vi "CSTK_Icon_Creator_Dialog.vi"() -> ()   [LabVIEW 2015, in "CSTK_Icon Creator.lvlib"]
uses:
  CSTK_Icon Creator.lvlib
  <vilib>/Utility/miscctls.llb/LVBoundsTypeDef.ctl
  <vilib>/picture/picture.llb/imagedata.ctl
  CSTK_Icon_Creator_Template.ctl
  user32.dll
panel:
  in  "Shutdown":bool
  in  "Minimize":bool
  in  "字体":enum16{"Small Fonts", "6px2bus"}(ring)
  in  "偏移":i8(slide) caption="0" scale=-16.0..16.0
  in  "LOGO":u16(ring)
  in  "保存图标按钮":bool
  in  "生成图标按钮":bool
  in  "主体背景色":u32(colorbox)=16777215
  in  "标题背景色":u32(colorbox)=16777215
  in  "字体颜色":u32(colorbox)
  in  "标题字符":string
  out "4#":picture
  out "3#":picture
  out "2#":picture
  out "1#":picture
  # "Icon Creator"
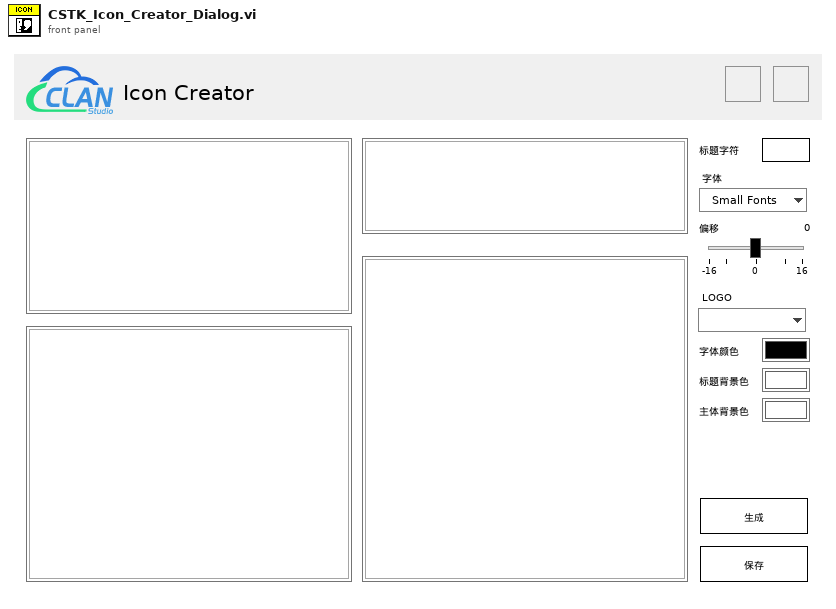
[diagram p1: front panel]
types:
  T1 = enum32{"Invalid", "Standard", "Closed", "Hidden", "Minimized", "Maximized"}
  T2 = typedef "imagedata.ctl" = cluster{"image type":i32, "image depth":i32, "image":u8[], "mask":u8[], "colors":u32[], "Rectangle":cluster{"left":i16, "top":i16, "right":i16, "bottom":i16}}
  T3 = typedef "LVBoundsTypeDef.ctl" = cluster{"Width":u32, "Height":u32}
  T4 = typedef "CSTK_Icon Creator.lvlib/CSTK_Icon_Creator_Template.ctl" = enum16{"1#", "2#", "3#", "4#", "Ctl"}
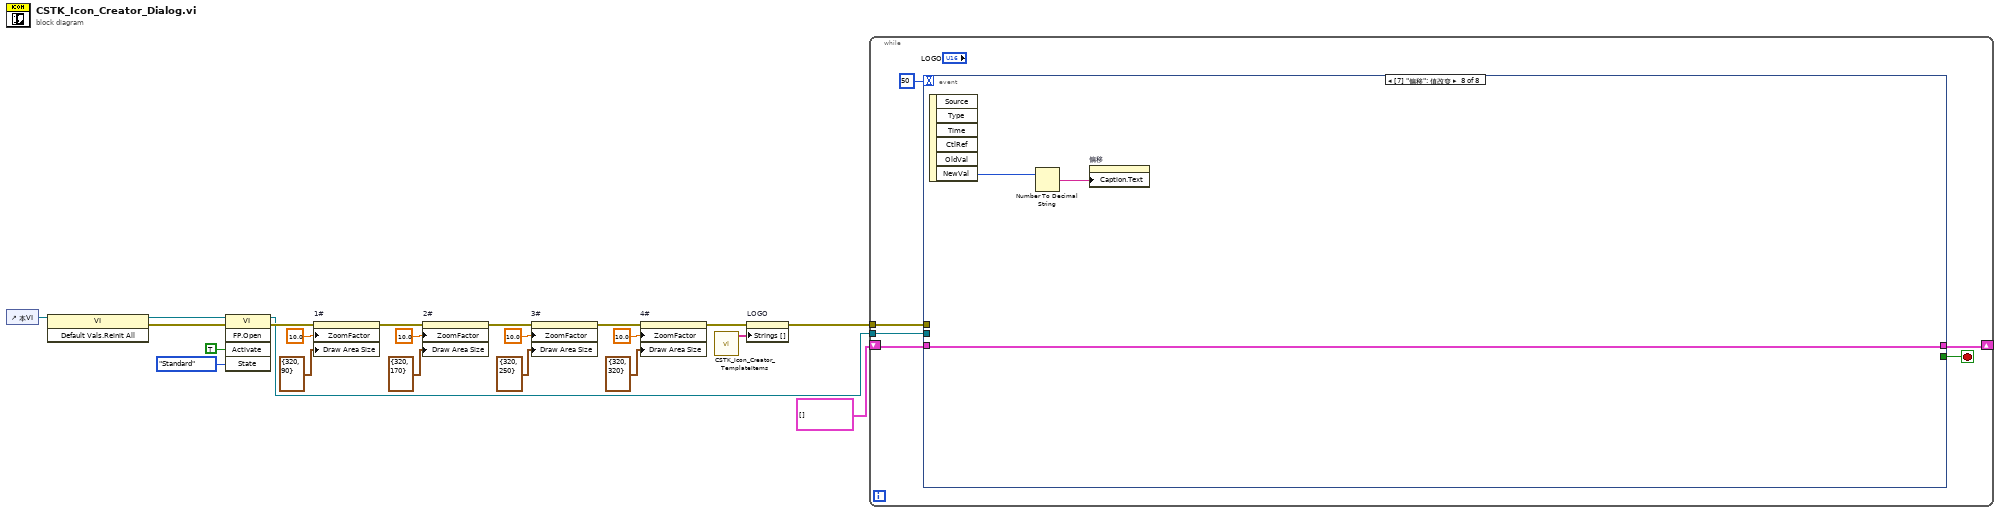
[diagram p0: block diagram]
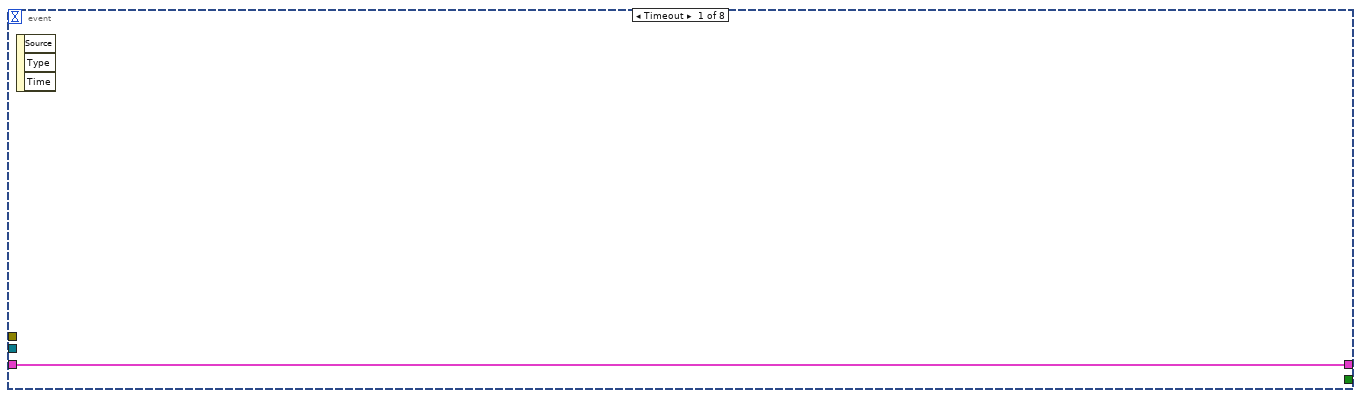
[diagram p2: hidden frame]
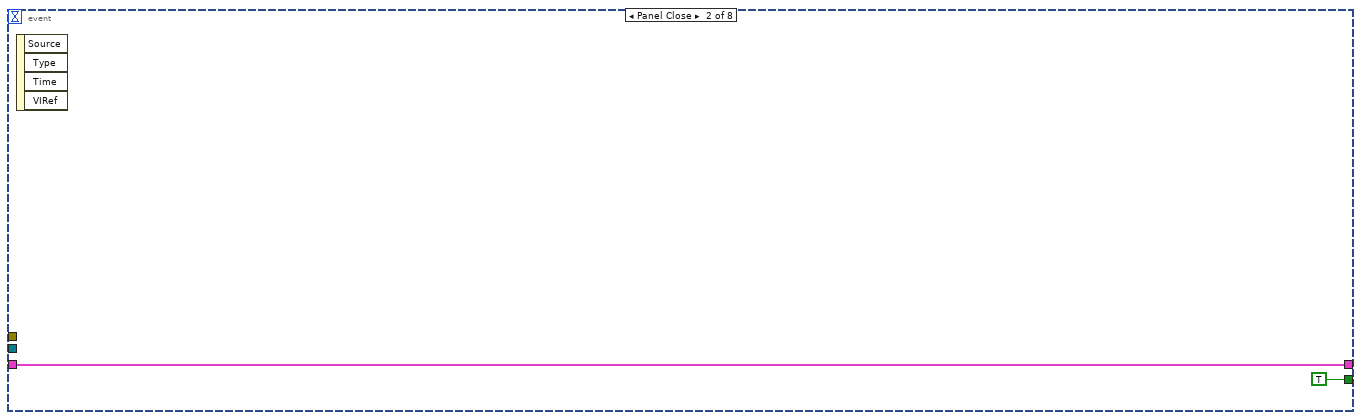
[diagram p3: hidden frame]
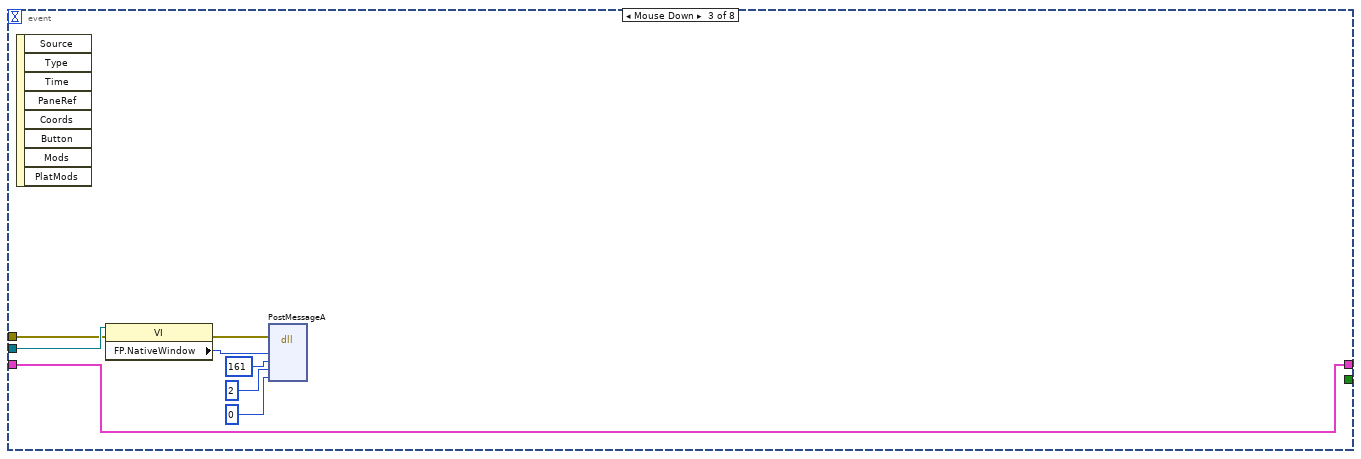
[diagram p4: hidden frame]
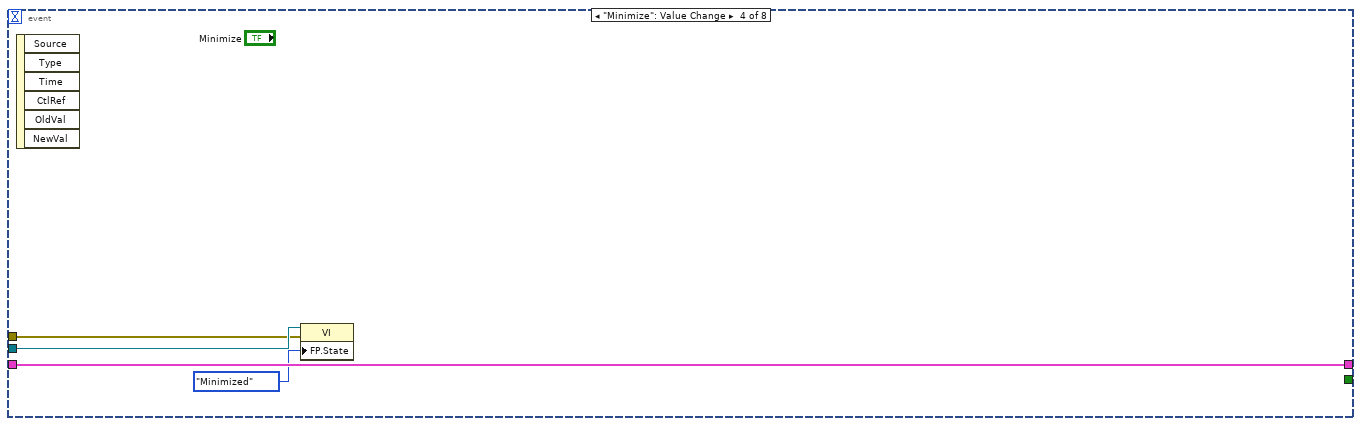
[diagram p5: hidden frame]
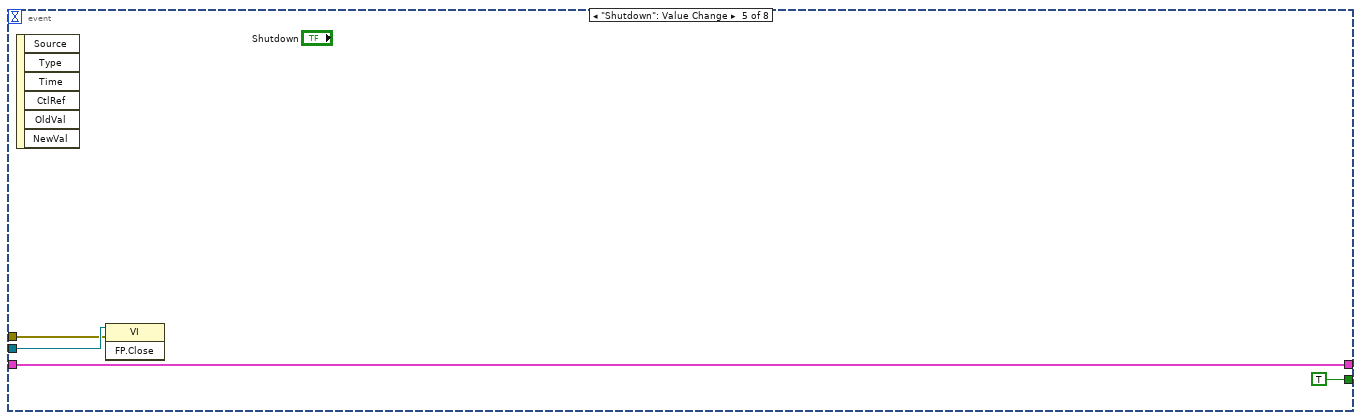
[diagram p6: hidden frame]
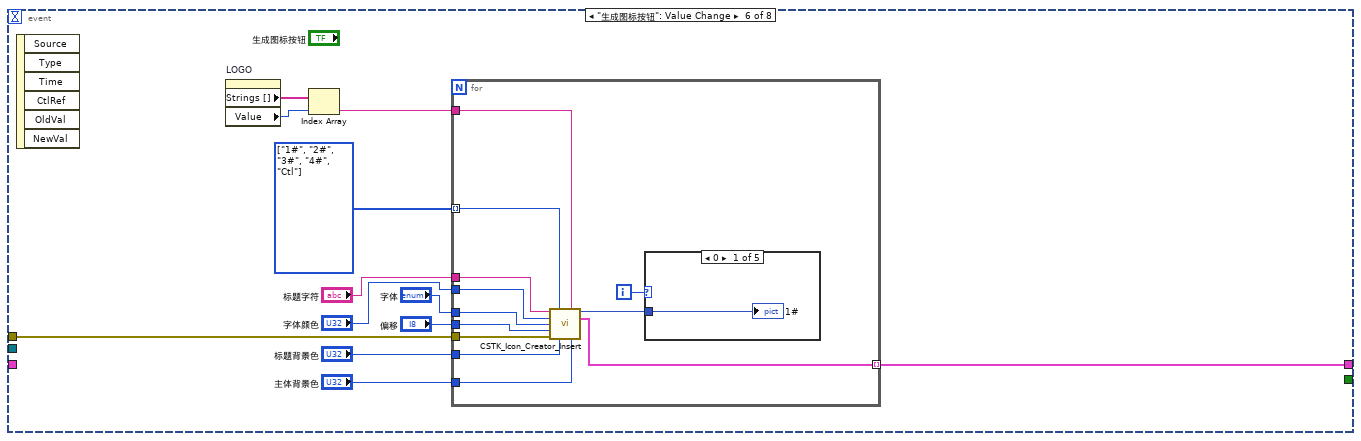
[diagram p7: hidden frame]
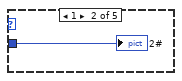
[diagram p8: hidden frame]
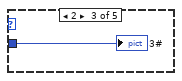
[diagram p9: hidden frame]
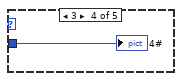
[diagram p10: hidden frame]
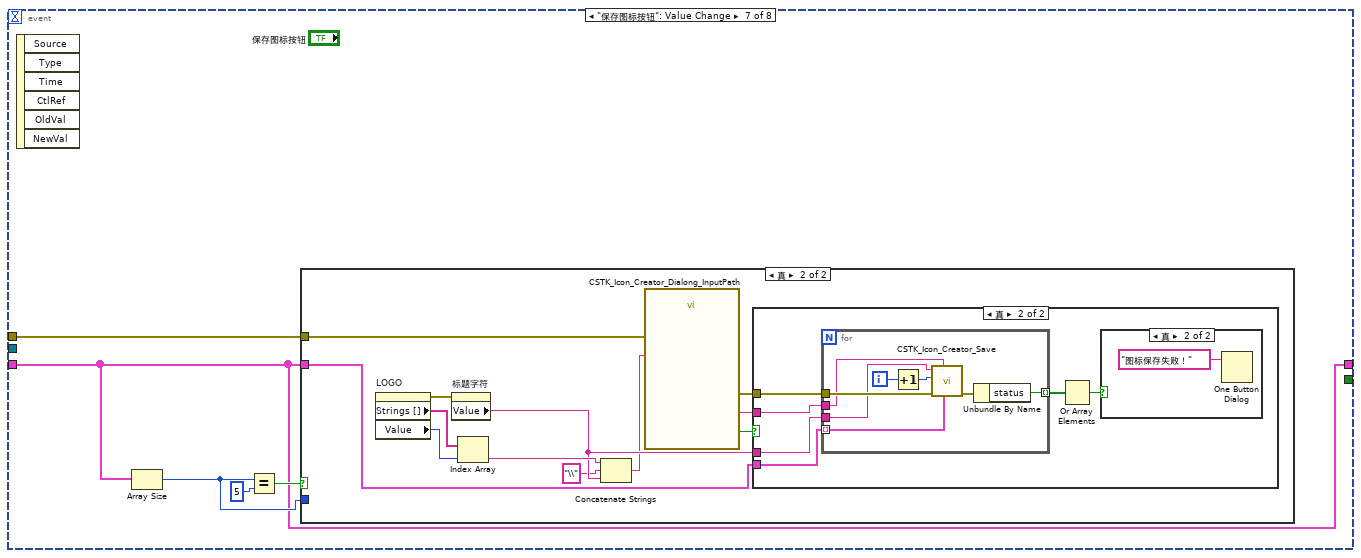
[diagram p12: hidden frame]
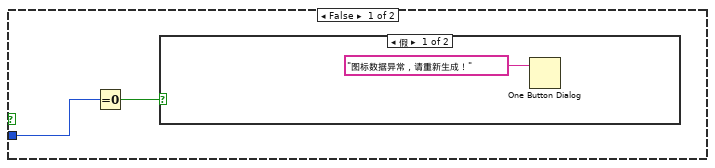
[diagram p13: hidden frame]
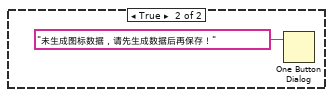
[diagram p14: hidden frame]
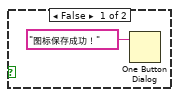
[diagram p16: hidden frame]
diagram:
  n1 = control-ref of="本VI"() -> (w10:refnum<vi>)
  n2 = invoke class="VI" method="Default Vals.Reinit All"(reference=w10) -> (reference out=w8:refnum<vi>, error out=w9:errorcluster)  [unwired: 2 in, 1 out]
  n3 = invoke class="VI" method="FP.Open"(reference=w8, error in=w9, "Activate"=TRUE ("激活？"), "State"=T1."Standard" ("状态")) -> (reference out=w1:refnum<vi>, error out=w7:errorcluster)  [unwired: 1 in, 3 out]
  n4 = property on="1#" class="Pict"(error in=w7, "ZoomFactor"=sgl 10.0 ("缩放因子"), "Draw Area Size"=T3 {"Width"=320, "Height"=90} ("绘图区域大小")) -> (error out=w18:errorcluster)  [unwired: 1 in, 1 out]
  n5 = property on="2#" class="Pict"(error in=w18, "ZoomFactor"=sgl 10.0 ("缩放因子"), "Draw Area Size"=T3 {"Width"=320, "Height"=170} ("绘图区域大小")) -> (error out=w15:errorcluster)  [unwired: 1 in, 1 out]
  n6 = property on="3#" class="Pict"(error in=w15, "ZoomFactor"=sgl 10.0 ("缩放因子"), "Draw Area Size"=T3 {"Width"=320, "Height"=250} ("绘图区域大小")) -> (error out=w12:errorcluster)  [unwired: 1 in, 1 out]
  n7 = property on="4#" class="Pict"(error in=w12, "ZoomFactor"=sgl 10.0 ("缩放因子"), "Draw Area Size"=T3 {"Width"=320, "Height"=320} ("绘图区域大小")) -> (error out=w3:errorcluster)  [unwired: 1 in, 1 out]
  n8 = call "CSTK_Icon_Creator_TemplateItems.vi"() -> ("TemplateItems"=w4:string[])  [unwired: 11 in]
  n9 = property on="LOGO" class="Ring (严格)"(error in=w3, "Strings []"=w4) -> (error out=w2:errorcluster)  [unwired: 1 in, 1 out]
  n10 = while {
    shift-right: [w26] -> _
    shift-left: T2[] [] ("图片数据") -> [w25]
    tunnel: w2 -> [w23]
    tunnel: w1 -> [w24]
    stop <- w28 stop-if-true
    n11 = event shown="[7] \"偏移\": 值改变" {
      selector: _ -> [_ _ _ _ _ _ _ _]
      dyn-events: _ -> [_ _ _ _ _ _ _ _]
      timeout: 50 -> [_ _ _ _ _ _ _ _]
      tunnel: [_ TRUE _ _ TRUE _ _ _] -> w28
      tunnel: [w29 w30 w39 w43 w47 w54 w77 w115] -> w26
      tunnel: w25 -> [w29 w30 w39 w43 w47 _ w77 w115]
      tunnel: w24 -> [_ _ w33 w41 w46 _ _ _]
      tunnel: w23 -> [_ _ w32 w40 w44 w48 w76 _]
      event Timeout {
        n12 = event-data() -> ()  [unwired: 1 in, 3 out]
      }
      event Panel Close {
        n13 = event-data() -> ()  [unwired: 1 in, 4 out]
      }
      event Mouse Down {
        n14 = event-data() -> ()  [unwired: 1 in, 8 out]
        n15 = property class="VI"(reference=w33, error in=w32) -> (error out=w34:errorcluster, "FP.NativeWindow"=w35:u64)  [unwired: 1 out]
        n16 = dll-call lib="user32.dll" fn="PostMessageA"(error in=w34, "hWnd"=w35, "Msg"=161, "wParam"=2, "IParam"=0 ("wParam")) -> ()  [unwired: 7 in, 2 out]
      }
      event "Minimize": Value Change {
        n17 = event-data() -> ()  [unwired: 1 in, 6 out]
        n18 = property class="VI"(reference=w41, error in=w40, "FP.State"=T1."Minimized" ("Front Panel Window:State")) -> ()  [unwired: 2 out]
      }
      event "Shutdown": Value Change {
        n19 = event-data() -> ()  [unwired: 1 in, 6 out]
        n20 = invoke class="VI" method="FP.Close"(reference=w46, error in=w44) -> ()  [unwired: 1 in, 3 out]
      }
      event "生成图标按钮": Value Change {
        w59 = T4[] [enum."1#", enum."2#", enum."3#", enum."4#", enum."Ctl"] items=["1#", "2#", "3#", "4#", "Ctl"] ("模板选择")
        n21 = event-data() -> ()  [unwired: 1 in, 6 out]
        n22 = property on="LOGO" class="Ring (严格)"() -> ("Strings []"=w50:string[], "Value"=w51:u16)  [unwired: 2 in, 2 out]
        n23 = Index Array(array=w50, index=w51) -> (element=w49:string)
        n24 = for {
          tunnel: w59 -> [w71] mode=indexing
          tunnel: "标题字符" -> [w64]
          tunnel: "字体颜色" -> [w63]
          tunnel: "标题背景色" -> [w70]
          tunnel: "主体背景色" -> [w69]
          tunnel: [w68] -> w54 mode=indexing
          tunnel: w49 -> [w65]
          tunnel: "偏移" -> [w62]
          tunnel: "字体" -> [w61]
          tunnel: w48 -> [w60]
          i -> [w67]
          n25 = call "CSTK_Icon_Creator_Insert.vi"("字符"=w64, "模板选择"=w71, "LOGO"=w65, "字体颜色"=w63, "字体"=w61, "水平偏移"=w62, "error in (no error)"=w60, "标题背景色"=w70, "主体背景色"=w69) -> ("图片"=w66:picture, "图片数据"=w68:T2)  [unwired: 4 in, 1 out]
          n26 = case shown="0" w67 {
            tunnel: w66 -> [w72 w73 w74 w75 _]
            frame 0 {
              "1#" <- w72
            }
            frame 1 {
              "2#" <- w73
            }
            frame 2 {
              "3#" <- w74
            }
            frame 3 {
              "4#" <- w75
            }
            frame Default {
            }
          }
        }
      }
      event "保存图标按钮": Value Change {
        n27 = event-data() -> ()  [unwired: 1 in, 6 out]
        n28 = Array Size(array=w77) -> (size(s)=w78:i32)
        n29 = Equal?(x=w78, y=5) -> (x = y?=w79:bool)
        n30 = case shown="真" w79 {
          tunnel: w78 -> [w82 _]
          tunnel: w77 -> [_ w96]
          tunnel: w76 -> [_ w85]
          frame False {
            n31 = Equal To 0?(x=w82) -> (x = 0?=w81:bool)
            n32 = case shown="假" w81 {
              frame False {
                n33 = One Button Dialog(message="图标数据异常，请重新生成！" ("消息")) -> ()  [unwired: 1 in, 1 out]
              }
              frame True {
                n34 = One Button Dialog(message="未生成图标数据，请先生成数据后再保存！" ("消息")) -> ()  [unwired: 1 in, 1 out]
              }
            }
          }
          frame True {
            n35 = property on="LOGO" class="Ring (严格)"() -> (error out=w90:errorcluster, "Strings []"=w91:string[], "Value"=w92:u16)  [unwired: 2 in, 1 out]
            n36 = property on="标题字符" class="Str"(error in=w90) -> ("Value"=w88:string)  [unwired: 1 in, 2 out]
            n37 = Index Array(array=w91, index=w92) -> (element=w89:string)
            n38 = Concatenate Strings(w89, "\\" ("字符串"), w88) -> (w86:string)
            n39 = call "CSTK_Icon_Creator_Dialong_InputPath.vi"("分类文件夹名输入"=w86, "error in (no error)"=w85) -> ("分类文件夹名输出"=w94:string, "确定"=w93:bool, "error out"=w95:errorcluster)  [unwired: 15 in]
            n40 = case shown="真" w93 {
              tunnel: w96 -> [_ w102]
              tunnel: w95 -> [_ w99]
              tunnel: w88 -> [_ w98]
              tunnel: w94 -> [_ w97]
              frame False {
              }
              frame True {
                n41 = for {
                  tunnel: w102 -> [w110] mode=indexing
                  tunnel: [w108] -> w101 mode=indexing
                  tunnel: w99 -> [w107]
                  tunnel: w98 -> [w106]
                  tunnel: w97 -> [w105]
                  i -> [w112]
                  n42 = Increment(x=w112) -> (x+1=w111:i32)
                  n43 = call "CSTK_Icon_Creator_Save.vi"("image data"=w110, "路径字符"=w105, "错误输入（无错误）"=w107, "序号"=w111, "标题字符"=w106) -> ("错误输出"=w109:errorcluster)  [unwired: 6 in]
                  n44 = Unbundle By Name(w109) -> ("status"=w108:bool)
                }
                n45 = Or Array Elements(Boolean array=w101) -> (logical OR=w100:bool)
                n46 = case shown="真" w100 {
                  frame False {
                    n47 = One Button Dialog(message="图标保存成功！" ("消息")) -> ()  [unwired: 1 in, 1 out]
                  }
                  frame True {
                    n48 = One Button Dialog(message="图标保存失败！" ("消息")) -> ()  [unwired: 1 in, 1 out]
                  }
                }
              }
            }
          }
        }
      }
      event "偏移": Value Change {
        n49 = event-data() -> ("NewVal"=w114:i8)  [unwired: 1 in, 5 out]
        n50 = Number To Decimal String(number=w114) -> (decimal integer string=w113:string)  [unwired: 1 in]
        n51 = property on="偏移" class="Slide (严格)"("Caption.Text"=w113) -> ()  [unwired: 2 in, 2 out]
      }
    }
  }
